vi "prepareVegMeal.vi"(8 "error in (no error)":errorcluster, 11 "MealBuilder in":refnum<class "MealBuilder.lvclass">) -> (0 "error out":errorcluster, 2 "Meal out":refnum<class "Meal.lvclass">, 3 "MealBuilder out":refnum<class "MealBuilder.lvclass">)   [LabVIEW 2018, in "MealBuilder.lvclass"]
uses:
  MealBuilder.lvclass
  Meal Class/Meal.lvclass
  VegBurger Class/VegBurger.lvclass
  C:/Users/fflores/Documents/LabVIEW-Open-Projects/LabIVEW OOP Design Patterns/Builder Pattern/Item Class/Item.lvclass
  Coke Class/Coke.lvclass
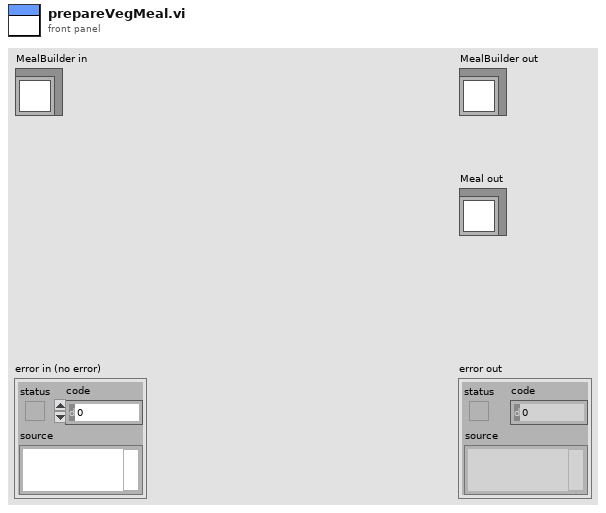
[diagram p1: front panel]
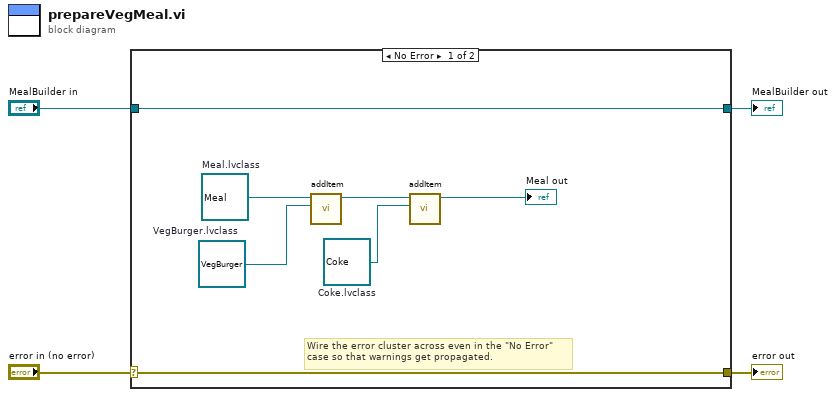
[diagram p0: block diagram]
diagram:
  n1 = case shown="No Error" "error in (no error)" {
    selector: "error in (no error)" -> [w10 w13]
    tunnel: [w10 w13] -> w3
    tunnel: [w11 w12] -> w1
    tunnel: "MealBuilder in" -> [w11 w12]
    frame No Error {
      w6 = refnum<class "Coke.lvclass"> refnum  # Coke.lvclass
      w7 = refnum<class "VegBurger.lvclass"> refnum  # VegBurger.lvclass
      w9 = refnum<class "Meal.lvclass"> refnum  # Meal.lvclass
      # "Wire the error cluster across even in the \"No Error\"\ncase so that warnings get propagated."
      n2 = call-dynamic "addItem.vi"("Item.lvclass"=w7, "Meal in"=w9) -> ("Meal out"=w8:refnum<class "Meal.lvclass">)  [unwired: 8 in, 1 out]
      n3 = call-dynamic "addItem.vi"("Item.lvclass"=w6, "Meal in"=w8) -> ("Meal out"=→"Meal out":refnum<class "Meal.lvclass">)  [unwired: 8 in, 1 out]
    }
    frame Error {
    }
  }
  "error out" <- w3
  "MealBuilder out" <- w1
